vi "getControlMatrixDH.vi"(8 "error in (no error)":errorcluster, 11 "DataHandler in":refnum<class "DataHandlerMYiTOPS.lvclass">) -> (0 "error out":errorcluster, 1 "List of ColHads":string[](array[string]), 2 "Array":string[][](array[string]), 3 "DataHandler out":refnum<class "DataHandlerMYiTOPS.lvclass">, 4 "Field Elements":string[](array[string]), 6 "List of ColHads 2":string[](array[string]))   [LabVIEW 2017, in "DataHandlerMYiTOPS.lvclass"]
uses:
  DataHandlerMYiTOPS.lvclass
  DataHandlerMYiTOPS.lvclass/DataHandlerMYiTOPS.ctl
  <vilib>/drjdpowell/SQLite Library/SQL Connection/Execute SQL.vi
  <vilib>/drjdpowell/SQLite Library/SQLite.lvlib
  <vilib>/drjdpowell/SQLite Library/SQL Connection/Connection.lvclass
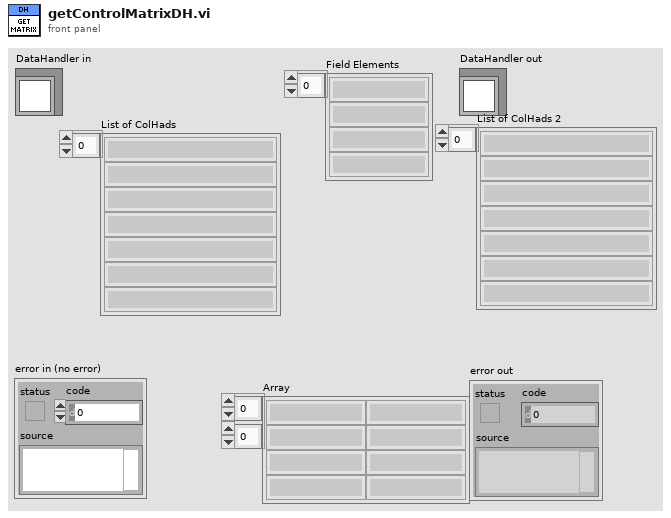
[diagram p1: front panel]
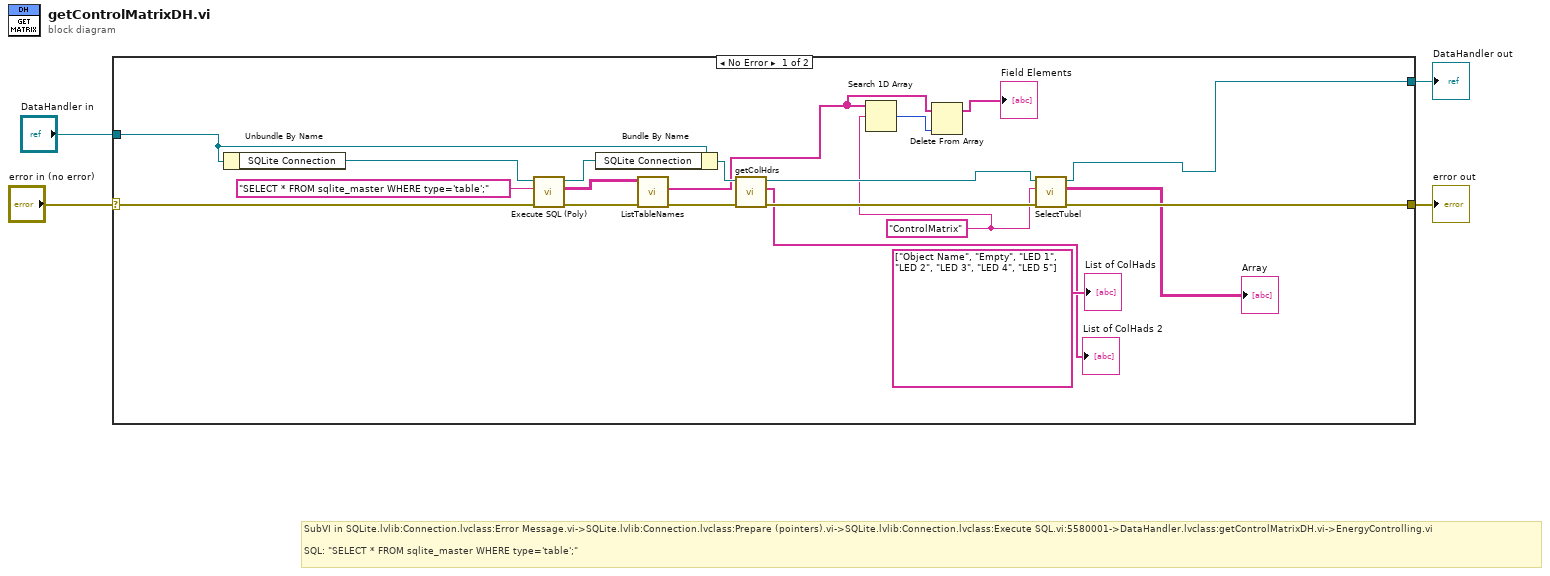
[diagram p0: block diagram]
diagram:
  # "SubVI in SQLite.lvlib:Connection.lvclass:Error Message.vi->SQLite.lvlib:Connection.lvclass:Prepare (pointers).vi->SQLite.lvlib:Connection.lvclass:Execute SQL.vi:5580001->DataHandler.lvclass:getControlMatrixDH.vi->EnergyControlling.vi\n\nSQL: \"SELECT * FROM sqlite_master WHERE type='table';\""
  n1 = case shown="No Error" "error in (no error)" {
    selector: "error in (no error)" -> [w18 w26]
    tunnel: [w24 w26] -> w3
    tunnel: [w23 w25] -> w1
    tunnel: "DataHandler in" -> [w17 w25]
    frame No Error {
      w8 = "ControlMatrix" ("element")
      n2 = Unbundle By Name(w17) -> ("SQLite Connection"=w19:refnum<class "Connection.lvclass">)
      n3 = call-poly <vilib>:"Execute SQL (Poly).vi"("error in (no error)"=w18, "SQL"="SELECT * FROM sqlite_master WHERE type='table';" ("String"), "SQLite Connection in"=w19) -> ("error out"=w22:errorcluster, "Result Set"=w21:string[][], "SQLite Connection out"=w16:refnum<class "Connection.lvclass">)  [unwired: 5 in, 1 out]
      n4 = Bundle By Name(cluster=w17, "SQLite Connection"=w16) -> (w13:refnum<class "DataHandlerMYiTOPS.lvclass">)
      n5 = call "ListTableNames.vi"("error in (no error)"=w22, "Result Set"=w21) -> ("error out"=w15:errorcluster, "Table Names"=w10:string[])  [unwired: 7 in, 1 out]
      n6 = call-dynamic "getColHdrs.vi"("error in (no error)"=w15, "DataHandler in"=w13) -> ("error out"=w14:errorcluster, "List of ColHads"=→"List of ColHads 2":string[], "DataHandler out"=w12:refnum<class "DataHandlerMYiTOPS.lvclass">)  [unwired: 7 in]
      n7 = Search 1D Array(1D array=w10, element=w8) -> (index of element=w11:i32)  [unwired: 1 in]
      n8 = Delete From Array(array=w10, index=w11) -> (array with subset deleted=→"Field Elements":string[])  [unwired: 1 in, 1 out]
      n9 = call-dynamic "SelectTubel.vi"("error in (no error)"=w14, "Unique Object Identifier"=w8, "DataHandler in"=w12) -> ("error out"=w24:errorcluster, "Array"=→"Array":string[][], "DataHandler out"=w23:refnum<class "DataHandlerMYiTOPS.lvclass">)  [unwired: 6 in]
      "List of ColHads" <- string[] ["Object Name", "Empty", "LED 1", "LED 2", "LED 3", "LED 4", "LED 5"] ("List of ColHads")
    }
    frame Error {
    }
  }
  "error out" <- w3
  "DataHandler out" <- w1
